vi "Digital input.vi"(8 "error in":errorcluster, 11 "DAQmx InPut Setting":T1) -> (0 "error out":errorcluster, 1 "Exit":bool)   [LabVIEW 2015]
uses:
  <vilib>/DAQmx/read.llb/DAQmx Read (Digital 1D Bool 1Chan 1Samp).vi
  <vilib>/DAQmx/create/channels.llb/DAQmx Create Channel (DI-Digital Input).vi
  Galobal variable_TI.vi
  <vilib>/DAQmx/miscellaneous.llb/DAQmx Fill In Error Info.vi
panel:
  out "Array":bool[](array[boolean])
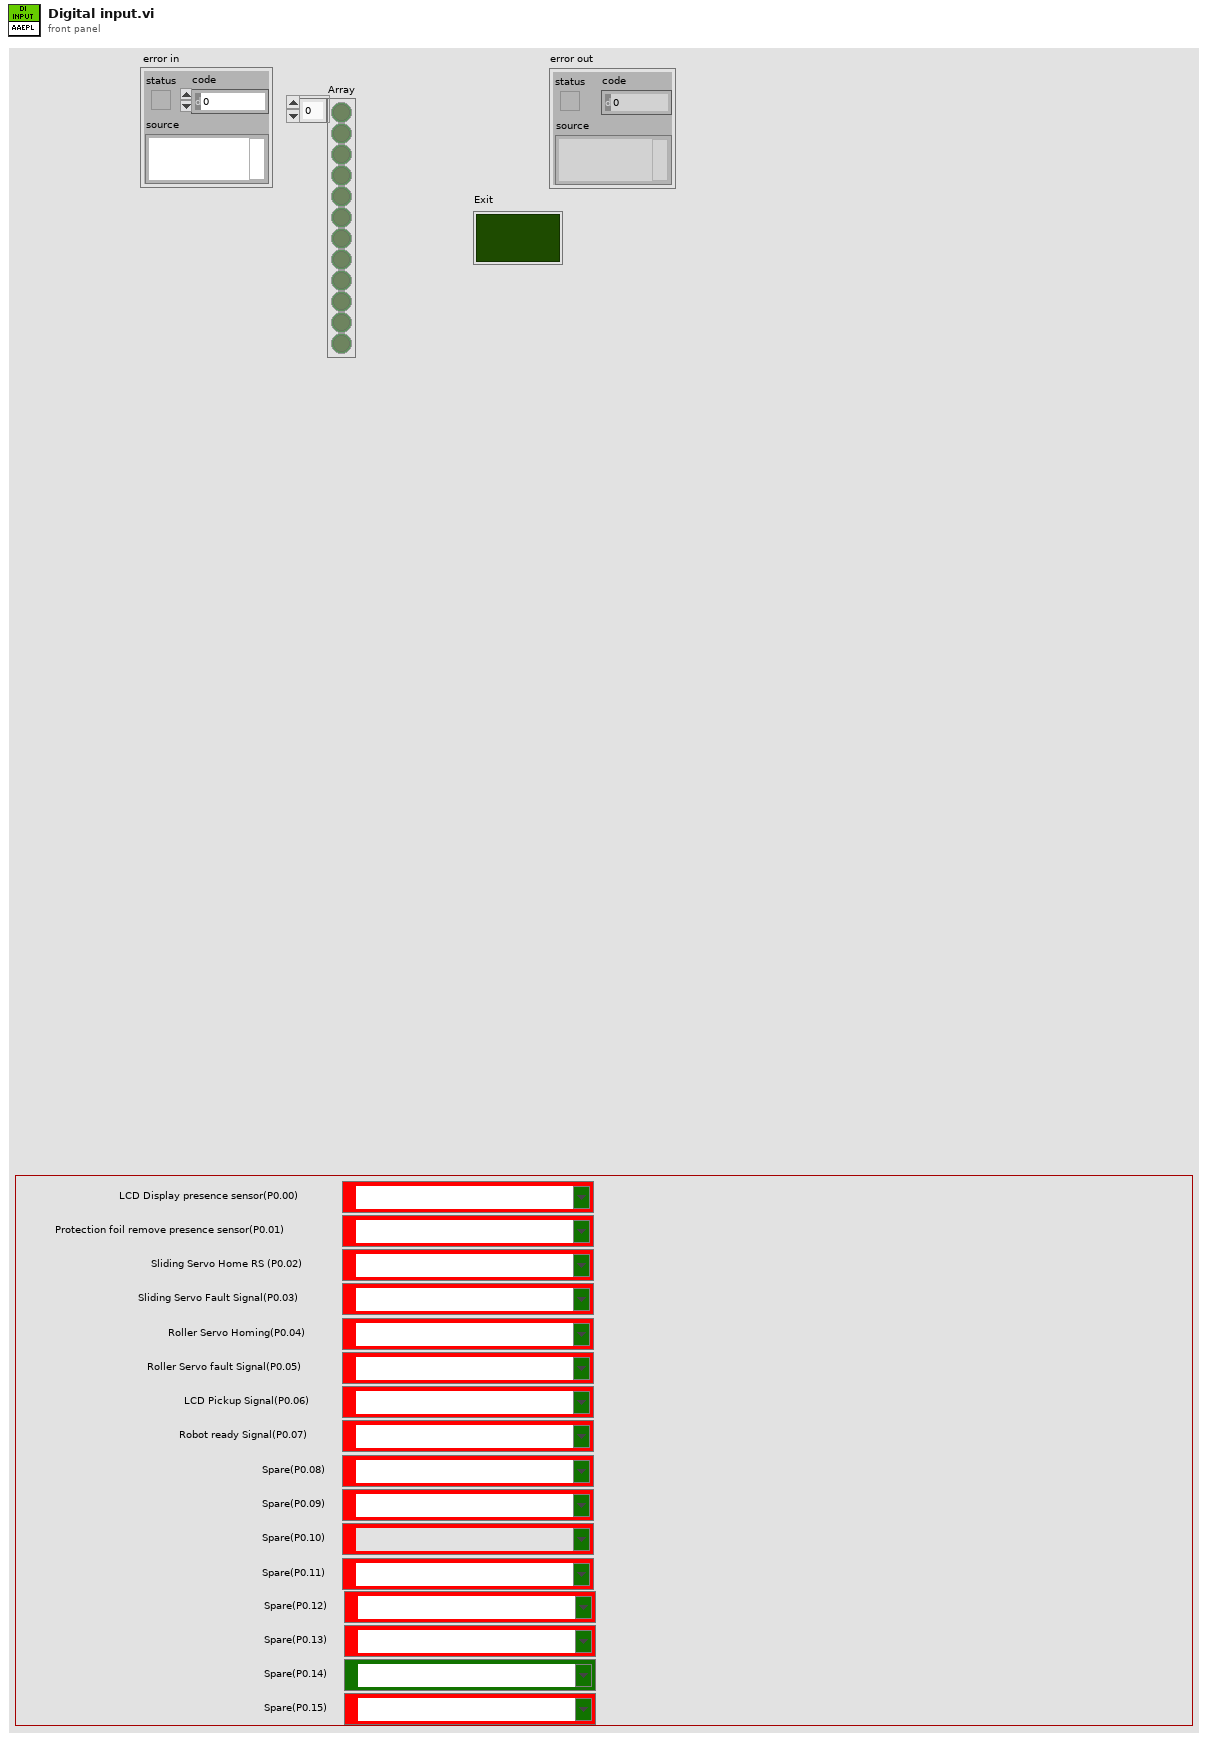
[diagram p1: front panel]
types:
  T1 = cluster{"DAQmx InPut_00":tag, "DAQmx InPut_01":tag, "DAQmx InPut_02":tag, "DAQmx InPut_03":tag, "DAQmx InPut_04":tag, "DAQmx InPut_05":tag, "DAQmx InPut_06":tag, "DAQmx InPut_07":tag, "DAQmx InPut_08":tag, "DAQmx InPut_09":tag, "DAQmx InPut_10":tag, "DAQmx InPut_11":tag, "DAQmx InPut_12":tag, "DAQmx InPut_13":tag, "DAQmx InPut_14":tag, "DAQmx InPut_15":tag}
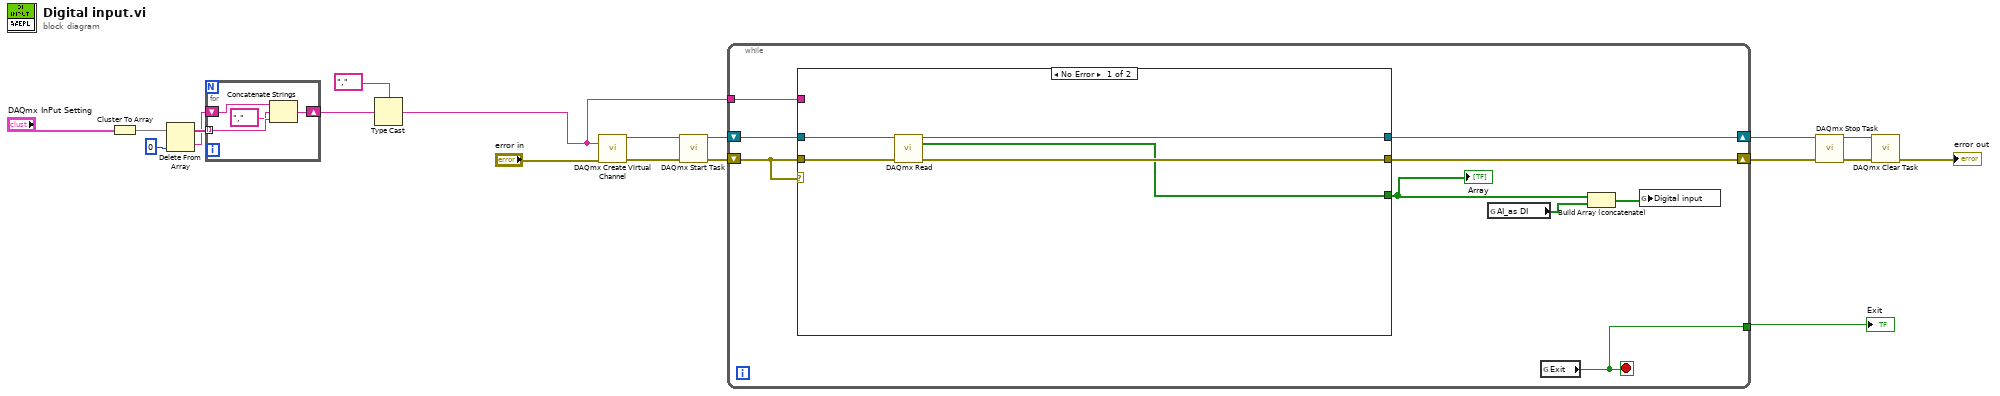
[diagram p0: block diagram]
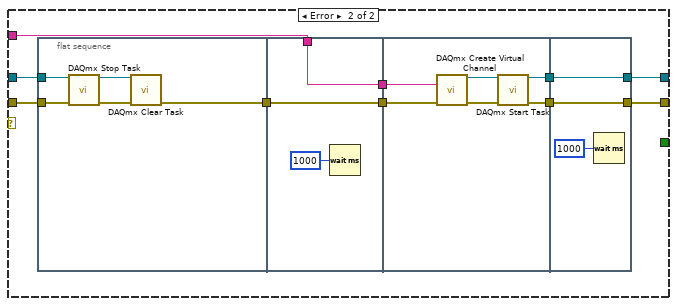
[diagram p2: hidden frame]
diagram:
  n1 = Cluster To Array(cluster="DAQmx InPut Setting") -> (array=w9:tag[])
  n2 = Delete From Array(array=w9, index=0) -> (deleted portion=w6:tag, array with subset deleted=w8:tag[])  [unwired: 1 in]
  n3 = for {
    tunnel: w8 -> [w22] mode=indexing
    shift-right: [w20] -> w4
    shift-left: w6 -> [w23]
    n4 = Concatenate Strings(w23, tag "," ("1."), w22) -> (w20:string)
  }
  n5 = Type Cast(type=tag "," ("1."), x=w4) -> (*(type *) &x=w3:tag)
  n6 = call-poly <vilib>:"DAQmx Create Virtual Channel.vi"("lines"=w3, "error in"="error in") -> ("task out"=w19:refnum<k21>, "error out"=w18:errorcluster)  [unwired: 3 in, 9 out]
  n7 = call <vilib>:"DAQmx Start Task.vi"("task/channels in"=w19, "error in"=w18) -> ("task out"=w16:refnum<k21>, "error out"=w17:errorcluster)  [unwired: 12 out]
  n8 = while {
    shift-right: [w32] -> w13
    shift-left: w17 -> [w31]
    shift-right: [w29] -> w12
    shift-left: w16 -> [w30]
    tunnel: w3 -> [w28]
    tunnel: [w26] -> w10
    stop <- w26 stop-if-true
    n9 = case shown="No Error" w31 {
      tunnel: w31 -> [w37 w46]
      tunnel: w30 -> [w36 w47]
      tunnel: [w35 w39] -> w32
      tunnel: [w34 w38] -> w29
      tunnel: w28 -> [_ w42]
      tunnel: [w33 _] -> w27
      frame No Error {
        n10 = call-poly <vilib>:"DAQmx Read.vi"("task/channels in"=w36, "error in"=w37) -> ("task out"=w34:refnum<k21>, "data"=w33:bool[], "error out"=w35:errorcluster)  [unwired: 1 in, 10 out]
      }
      frame Error {
        n11 = flat-sequence {
          tunnel: w47 -> [w50]
          tunnel: w46 -> [w49]
          tunnel: [w48] -> w45
          tunnel: w45 -> [w54]
          tunnel: [w54] -> w44
          tunnel: [w53] -> w43
          tunnel: w42 -> [w53]
          tunnel: w44 -> [w59]
          tunnel: w43 -> [w58]
          tunnel: [w57] -> w41
          tunnel: [w56] -> w40
          tunnel: w41 -> [w64]
          tunnel: w40 -> [w63]
          tunnel: [w64] -> w39
          tunnel: [w63] -> w38
          frame #0 {
            n12 = call <vilib>:"DAQmx Stop Task.vi"("task/channels in"=w50, "error in"=w49) -> ("task out"=w51:refnum<k21>, "error out"=w52:errorcluster)  [unwired: 12 in]
            n13 = call <vilib>:"DAQmx Clear Task.vi"("task in"=w51, "error in"=w52) -> ("error out"=w48:errorcluster)  [unwired: 13 in]
          }
          frame #1 {
            n14 = Wait (ms)(milliseconds to wait=u32 1000) -> ()  [unwired: 1 out]
          }
          frame #2 {
            n15 = call-poly <vilib>:"DAQmx Create Virtual Channel.vi"("lines"=w58, "error in"=w59) -> ("task out"=w60:refnum<k21>, "error out"=w61:errorcluster)  [unwired: 3 in, 9 out]
            n16 = call <vilib>:"DAQmx Start Task.vi"("task/channels in"=w60, "error in"=w61) -> ("task out"=w56:refnum<k21>, "error out"=w57:errorcluster)  [unwired: 12 out]
          }
          frame #3 {
            n17 = Wait (ms)(milliseconds to wait=u32 1000) -> ()  [unwired: 1 out]
          }
        }
      }
    }
    "Array" <- w27
    n18 = global read "Galobal variable_TI.vi" "AI_as DI"() -> (w24:bool[])
    n19 = global read "Galobal variable_TI.vi" "Exit"() -> (w26:bool)
    n20 = Build Array (concatenate)(w27, w24) -> (w25:bool[])
    n21 = global write "Galobal variable_TI.vi" "Digital input"(w25) -> ()
  }
  "Exit" <- w10
  n22 = call <vilib>:"DAQmx Stop Task.vi"("task/channels in"=w12, "error in"=w13) -> ("task out"=w14:refnum<k21>, "error out"=w15:errorcluster)  [unwired: 12 in]
  n23 = call <vilib>:"DAQmx Clear Task.vi"("task in"=w14, "error in"=w15) -> ("error out"=→"error out":errorcluster)  [unwired: 13 in]
